vi "Convert NaN to 0.vi"() -> ()   [LabVIEW 2011]
panel:
  out "Converted":dbl
  in  "Input":dbl
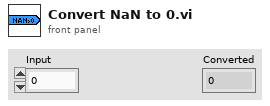
[diagram p1: front panel]
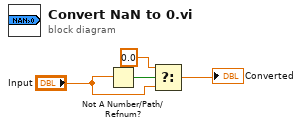
[diagram p0: block diagram]
diagram:
  n1 = Not A Number/Path/Refnum?(number/path/refnum="Input") -> (NaN/Path/Refnum?=w4:bool)
  n2 = Select(t=0.0, s=w4, f="Input") -> (s? t:f=→"Converted":dbl)
